vi "MoveFileToArchive.vi"(8 "error in (no error)":errorcluster, 10 "Source File":path, 11 "USB root":path) -> (0 "error out":errorcluster)   [LabVIEW 2017, in "USBDrive.lvlib"]
uses:
  <vilib>/addons/InsightCM/Devices/Shared/Common/USBDrive/USBDrive.lvlib
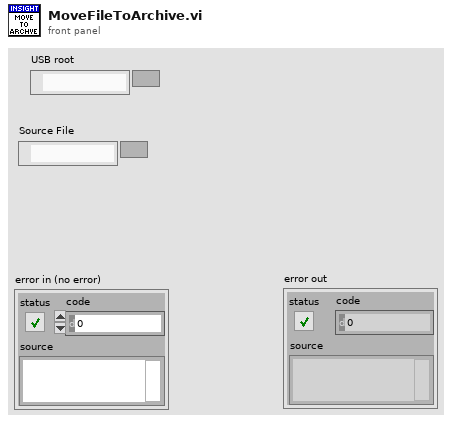
[diagram p1: front panel]
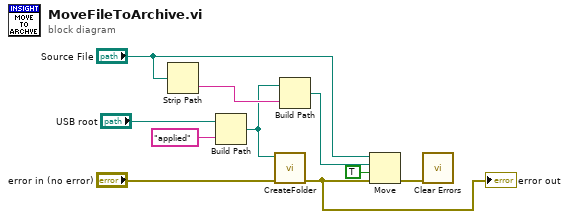
[diagram p0: block diagram]
diagram:
  n1 = Strip Path(path="Source File") -> (name=w8:string)  [unwired: 1 out]
  n2 = Build Path(base path="USB root", name or relative path="applied") -> (appended path=w1:path)
  n3 = call <vilib>:"CreateFolder.vi"("error in (no error)"="error in (no error)", "folder"=w1) -> ("error out"=w2:errorcluster)  [unwired: 8 in, 1 out]
  "error out" <- w2
  n4 = Build Path(base path=w1, name or relative path=w8) -> (appended path=w7:path)
  n5 = Move(source path="Source File", error in=w2, 9:TRUE ("overwrite (F)"), 10:w7) -> (error out=w4:errorcluster)  [unwired: 1 in, 2 out]
  n6 = call <vilib>:"Clear Errors.vi"("error in (no error)"=w4) -> ()  [unwired: 5 in, 2 out]
